vi "Command_Actuate_Disc_Intake.vi"(7 "Startup":bool, 9 "Wait(ms)":u32) -> (2 "Actuate":bool, 4 "Reinit":bool, 6 "Completed":bool)   [LabVIEW 2018]
uses:
  Autonomous Utilities/Command_Execution_State.ctl
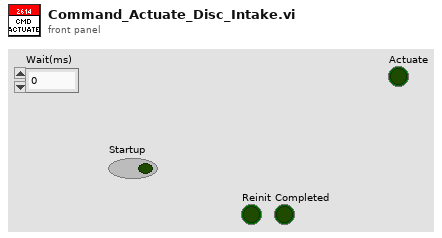
[diagram p1: front panel]
types:
  T1 = typedef "Command_Execution_State.ctl" = enum16{"Initialize", "Execute", "Finish"}
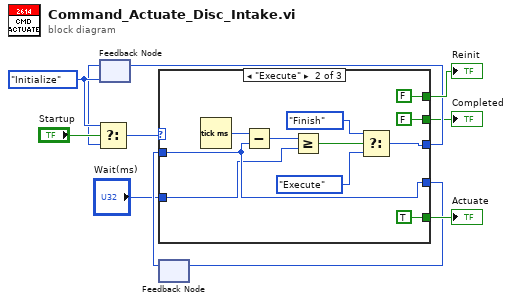
[diagram p0: block diagram]
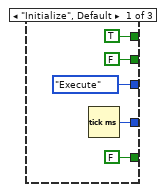
[diagram p2: hidden frame]
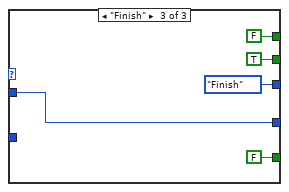
[diagram p3: hidden frame]
diagram:
  w9 = Command_Execution_State."Initialize" ("Play State")
  n1 = feedback #1(w9) -> (w8:T1)
  n2 = Select(t=w9, s="Startup", f=w8) -> (s? t:f=w10:T1)
  n3 = feedback #2() -> (w2:u32)  [unwired: 1 in]
  n4 = case shown="\"Execute\"" w10 {
    tunnel: [TRUE FALSE FALSE] -> w7
    tunnel: [FALSE TRUE FALSE] -> w4
    tunnel: [Command_Execution_State."Execute" ("Play State") w22 Command_Execution_State."Finish" ("Play State")] -> w6
    tunnel: [FALSE FALSE TRUE] -> w5
    tunnel: [w12 w23 w28] -> w3
    tunnel: w2 -> [_ w23 w28]
    tunnel: "Wait(ms)" -> [_ w17 _]
    frame "Initialize", Default {
      n5 = Tick Count (ms)() -> (millisecond timer value=w12:u32)
    }
    frame "Execute" {
      n6 = Tick Count (ms)() -> (millisecond timer value=w24:u32)
      n7 = Subtract(x=w24, y=w23) -> (x-y=w18:u32)
      n8 = Greater Or Equal?(x=w18, y=w17) -> (x >= y?=w19:bool)
      n9 = Select(t=Command_Execution_State."Finish" ("Play State"), s=w19, f=Command_Execution_State."Execute" ("Play State")) -> (s? t:f=w22:T1)
    }
    frame "Finish" {
    }
  }
  "Reinit" <- w7
  "Completed" <- w5
  "Actuate" <- w4
  n10 = feedback-in #1(w6) -> ()
  n11 = feedback-in #2(w3) -> ()
